vi "verify #frames.vi"(8 "error in (no error)":errorcluster, 11 "Simulated_CCD_Camera in":refnum<class "Sim_CCD.lvclass">) -> (0 "error out":errorcluster, 3 "Simulated_CCD_Camera out":refnum<class "Sim_CCD.lvclass">)   [LabVIEW 2018, in "Sim_CCD.lvclass"]
doc: "Verify the related parameters of the camera\n\nThere are some parameters of the camera operation mode that depend on the value provided for another parameter. This function verifies if these parameters are in agreement."
uses:
  Sim_CCD.lvclass
  Sim_CCD.lvclass/Sim_CCD.ctl
  <vilib>/ErrorRing/Error Ring.xnode
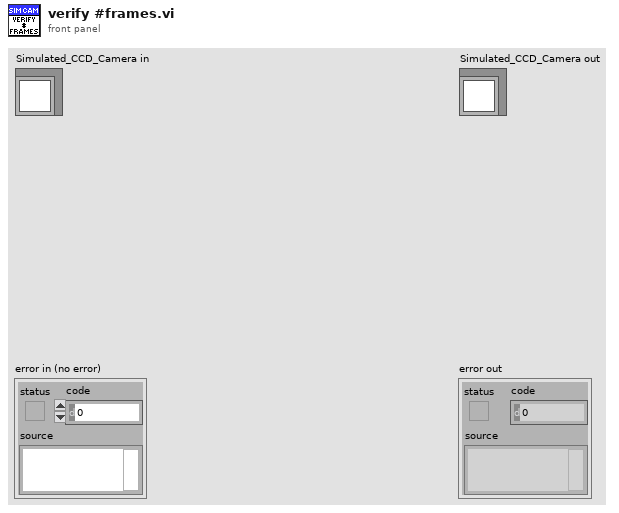
[diagram p1: front panel]
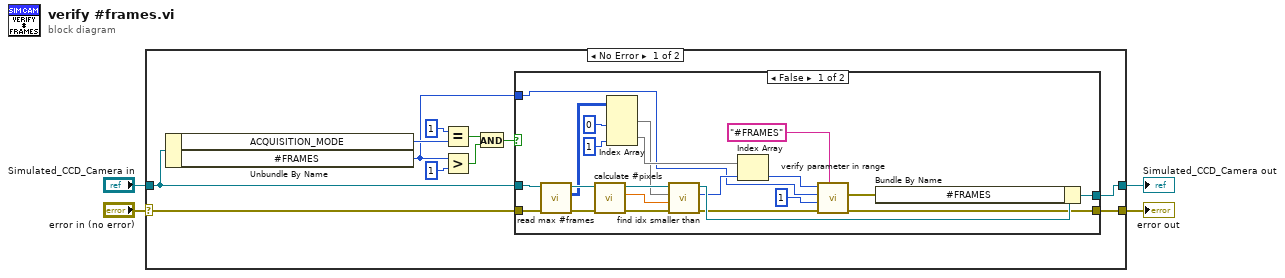
[diagram p0: block diagram]
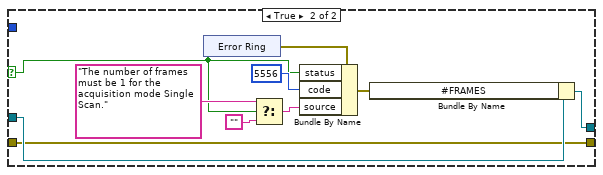
[diagram p2: hidden frame]
diagram:
  n1 = case shown="No Error" "error in (no error)" {
    selector: "error in (no error)" -> [w11 w50]
    tunnel: [w8 w50] -> w3
    tunnel: [w9 w49] -> w1
    tunnel: "Simulated_CCD_Camera in" -> [w10 w49]
    frame No Error {
      n2 = Unbundle By Name(w10) -> ("ACQUISITION_MODE"=w6:u16, "#FRAMES"=w5:u32)
      n3 = Equal?(x=u16 1, y=w6) -> (x = y?=w13:bool)
      n4 = Greater?(x=w5, y=1) -> (0:w14:bool)
      n5 = And(x=w13, y=w14) -> (x .and. y?=w7:bool)
      n6 = case shown="False" w7 {
        selector: w7 -> [_ w38]
        tunnel: [w29 w45] -> w9
        tunnel: w10 -> [w36 w46]
        tunnel: w11 -> [w37 w44]
        tunnel: [w16 w44] -> w8
        tunnel: w5 -> [w20 _]
        frame False {
          n7 = call "read max #frames.vi"("error in (no error)"=w37, "Simulated_CCD_Camera in"=w36) -> ("error out"=w35:errorcluster, "max #pix"=w33:i64[][], "Simulated_CCD_Camera out"=w34:refnum<class "Sim_CCD.lvclass">)  [unwired: 7 in]
          n8 = call "calculate #pixels.vi"("error in (no error)"=w35, "Simulated Camera in"=w34) -> ("error out"=w28:errorcluster, "#pixels"=w24:dbl, "Simulated Camera out"=w26:refnum<class "Sim_CCD.lvclass">)  [unwired: 7 in]
          n9 = Index Array(array=w33, index (col) #1=0 ("disabled index (col)"), index (col) #2=1 ("disabled index (col)")) -> (element #1=w25:i64[], element #2=w30:i64[])  [unwired: 2 in]
          n10 = call "find idx smaller than.vi"("error in (no error)"=w28, "Numeric"=w24, "Array"=w25, "Simulated Camera in"=w26) -> ("error out"=w17:errorcluster, "index"=w23:i32, "Simulated Camera out"=w27:refnum<class "Sim_CCD.lvclass">)  [unwired: 5 in]
          n11 = Index Array(array=w30, index=w23) -> (element=w19:i64)
          n12 = call "verify parameter in range.vi"("parameter name"="#FRAMES", "error in (no error)"=w17, "lower limit"=1, "value"=w20, "upper limit"=w19) -> ("error out"=w16:errorcluster, "verific error"=w18:errorcluster)  [unwired: 5 in]
          n13 = Bundle By Name(cluster=w27, "#FRAMES"=w18) -> (w29:refnum<class "Sim_CCD.lvclass">)
        }
        frame True {
          n14 = xnode "Error Ring"() -> ("error out"=w47:errorcluster)
          n15 = Select(t="The number of frames must be 1 for the acquisition mode Single Scan.", s=w38, f="") -> (s? t:f=w39:string)
          n16 = Bundle By Name(cluster=w47, "status"=w38, "code"=5556, "source"=w39) -> (w43:errorcluster)
          n17 = Bundle By Name(cluster=w46, "#FRAMES"=w43) -> (w45:refnum<class "Sim_CCD.lvclass">)
        }
      }
    }
    frame Error {
    }
  }
  "error out" <- w3
  "Simulated_CCD_Camera out" <- w1
